vi "Robot Global Data.vi"() -> ()   [LabVIEW 2018]
doc: "This global VI can contain as many global variables as you need. Place a control on the panel, give it a good name. To read or write to it from a VI, drag the icon to the diagram of that VI. You can also drag from the project. Click on the node to change which global you access. You shouldn't have multiple locations writing to a global or it will cause a race-condition."
uses:
  <vilib>/Rock Robotics/WPI/DriverStation/WPI_DriverStationRobotMode2.ctl
panel:
  in  "Pivot encoder counts":dbl=2048.0
  in  "Drive Motor Controller Type":T1(ring)=enum."Talon SRX Brushed"
  in  "Steer Encoder Values":dbl[](array[numeric])
  out "Yaw Angle":dbl
  out "Enable Steering":bool
  in  "Wheel Speeds":dbl[](array[numeric])
  in  "New Wheel Angles":dbl[](array[numeric])
  in  "Driver Joysticks?":T2(ring)
  in  "z target":dbl
  in  "y target":dbl
  in  "x target":dbl
  in  "Y Velocity":dbl
  in  "X Velocity":dbl
  in  "Reset Encoders":bool
  in  "Y Distance":dbl
  in  "X Distance":dbl
  in  "z":dbl
  in  "y":dbl
  in  "x":dbl
  in  "Robot Mode":T3
  # "Swerve Drive Controls"
  # "Enum Controls"
  # "Boolean Controls"
  # "Double Precision Controls"
  # "4096 for CTRE encoder\n2048 for Lamprey encoder"
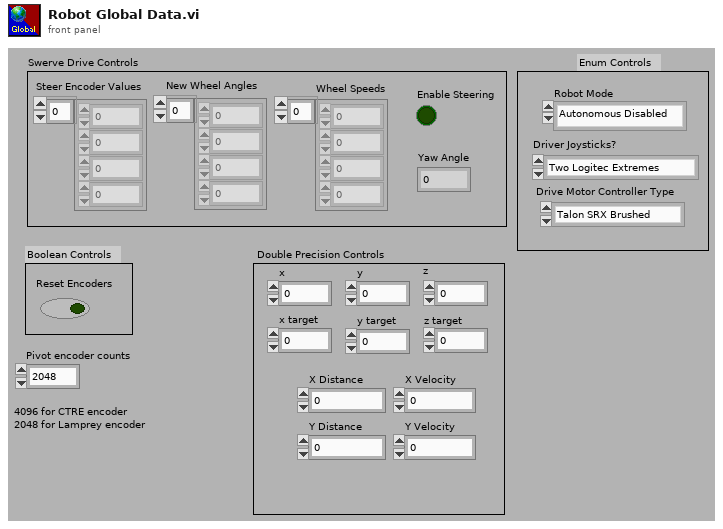
[diagram p1: front panel]
types:
  T1 = enum16{"Sparkmax Brushless", "Talon SRX Brushed"}
  T2 = enum16{"Two Logitec Extremes", "Dual Action Logitec", "Interlink"}
  T3 = typedef "WPI_DriverStationRobotMode2.ctl" = enum16{"Autonomous Disabled", "Autonomous Enabled", "Teleop Disabled", "Teleop Enabled", "Disconnected", "Finish", "Test Disabled", "Test Enabled", "Emergency Stopped"}
diagram:
